vi "Mediciones2.vi"() -> ()   [LabVIEW 2017]
panel:
  in  "Alto":dbl
  in  "Ancho":dbl
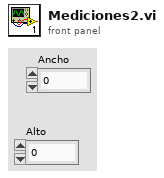
[diagram p1: front panel]
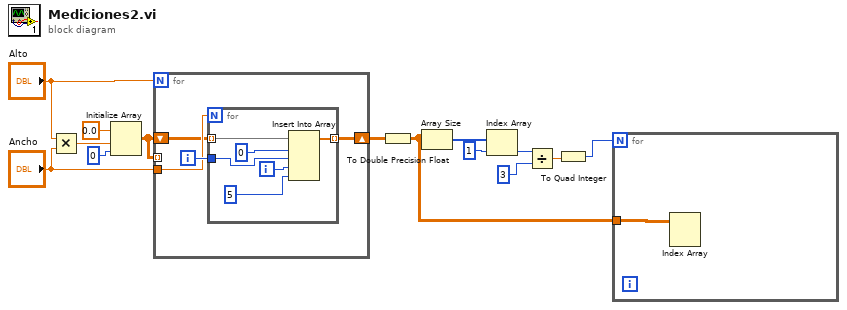
[diagram p0: block diagram]
diagram:
  n1 = Multiply(x="Alto", y="Ancho") -> (x*y=w12:dbl)
  n2 = Initialize Array(0.0, w12, 0) -> (w10:dbl[][])
  n3 = for {
    N: "Alto" -> [_]
    tunnel: "Ancho" -> [w17]
    tunnel: w10 -> [_] mode=indexing
    shift-right: [w15] -> w8
    shift-left: w10 -> [w16]
    i -> [w18]
    n4 = for {
      N: w17 -> [_]
      tunnel: w16 -> [w23] mode=indexing
      tunnel: [w22] -> w15 mode=indexing
      tunnel: w18 -> [w24]
      i -> [w20]
      n5 = Insert Into Array(array=w23, index=0, new element #1=w24, new element #2=w20, new element #3=5) -> (w22:dbl[])
    }
  }
  n6 = To Double Precision Float(number=w8) -> (double precision float=w1:dbl[][])
  n7 = Array Size(array=w1) -> (size(s)=w7:i32[])
  n8 = Index Array(array=w7, index=1) -> (element=w5:i32)
  n9 = Divide(x=w5, y=3) -> (x/y=w3:dbl)
  n10 = To Quad Integer(1:w3) -> (0:w2:i64)
  n11 = for {
    N: w2 -> [_]
    tunnel: w1 -> [w25]
    n12 = Index Array(array=w25) -> ()  [unwired: 2 in, 1 out]
  }
